vi "clear screen.vi"(4 "error in":errorcluster, 6 "Display in 2":string[][](array[string]), 7 "result string":string) -> (0 "error out":errorcluster, 1 "Screen Cleared":bool, 2 "Display in":string[][](array[string]), 3 "String":string)   [LabVIEW 2018]
uses:
  <vilib>/regexp/Match Regular Expression.xnode
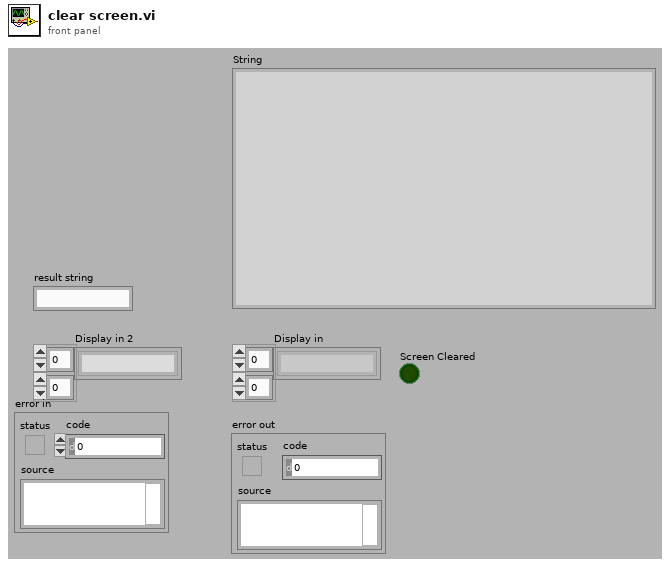
[diagram p1: front panel]
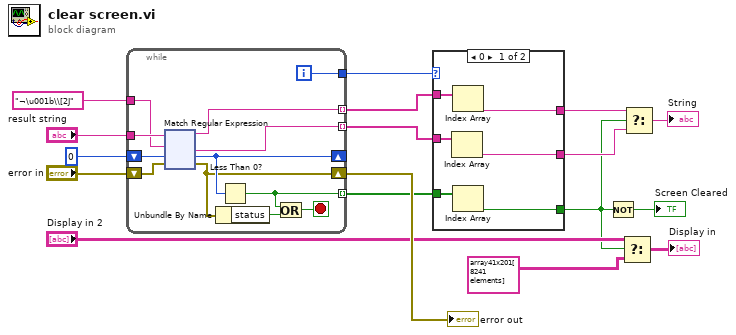
[diagram p0: block diagram]
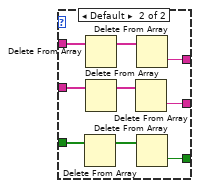
[diagram p2: hidden frame]
diagram:
  n1 = while {
    tunnel: "result string" -> [w29]
    tunnel: [w18] -> w3 mode=indexing
    tunnel: "¬\u001b\\[2J" ("regular expression") -> [w28]
    tunnel: [w26] -> w9 mode=indexing
    tunnel: [w25] -> w7 mode=indexing
    shift-right: [w21] -> w17
    shift-left: "error in" -> [w27]
    shift-right: [w24] -> _
    shift-left: 0 ("offset past match") -> [w23]
    tunnel: [w22] -> w4
    i -> [w22]
    stop <- w19 stop-if-true
    n2 = xnode "Match Regular Expression"("input string"=w29, "regular expression"=w28, "offset (0)"=w23, "error in"=w27) -> ("before match"=w26:string, "after match"=w25:string, "offset past match"=w24:i32, "error out"=w21:errorcluster)  [unwired: 2 in, 1 out]
    n3 = Unbundle By Name(w21) -> ("status"=w20:bool)
    n4 = Less Than 0?(x=w24) -> (x < 0?=w18:bool)
    n5 = Or(x=w18, y=w20) -> (x .or. y?=w19:bool)
  }
  "error out" <- w17
  n6 = case shown="0" w4 {
    tunnel: w9 -> [w146 w155]
    tunnel: [w143 w148] -> w8
    tunnel: w7 -> [w144 w154]
    tunnel: [w145 w149] -> w6
    tunnel: w3 -> [w142 w153]
    tunnel: [w141 w147] -> w2
    frame 0 {
      n7 = Index Array(array=w144) -> (element=w143:string)  [unwired: 1 in]
      n8 = Index Array(array=w146) -> (element=w145:string)  [unwired: 1 in]
      n9 = Index Array(array=w142) -> (element=w141:bool)  [unwired: 1 in]
    }
    frame Default {
      n10 = Delete From Array(array=w153) -> (array with subset deleted=w151:bool[])  [unwired: 2 in, 1 out]
      n11 = Delete From Array(array=w155) -> (array with subset deleted=w152:string[])  [unwired: 2 in, 1 out]
      n12 = Delete From Array(array=w154) -> (array with subset deleted=w150:string[])  [unwired: 2 in, 1 out]
      n13 = Delete From Array(array=w150) -> (deleted portion=w148:string)  [unwired: 2 in, 1 out]
      n14 = Delete From Array(array=w152) -> (deleted portion=w149:string)  [unwired: 2 in, 1 out]
      n15 = Delete From Array(array=w151) -> (deleted portion=w147:bool)  [unwired: 2 in, 1 out]
    }
  }
  n16 = Not(x=w2) -> (.not. x?=→"Screen Cleared":bool)
  n17 = Select(t="Display in 2", s=w2, f=string[][] array41x201[8241 elements] ("Display in")) -> (s? t:f=→"Display in":string[][])
  n18 = Select(t=w6, s=w2, f=w8) -> (s? t:f=→"String":string)
